vi "LinearQuadraticRegulator_LatencyCompensate.vi"(8 "InputDelay_Seconds":dbl, 9 "dT_Seconds":dbl, 10 "Plant":T1, 11 "in LinearQuadraticRegulator":T3) -> (0 "Error":bool, 3 "out LinearQuadraticRegulator":T3, 4 "ExponentNotRational":bool)   [LabVIEW 2019, in "Trajectory_Library.lvlib"]
doc: "Adjusts LQR controller gain to compensate for a pure time delay in the input.\n \nLinear-Quadratic regulator controller gains tend to be aggressive. If sensor measurements are time-delayed too long, the LQR may be unstable. However, if we know the amount of delay, we can compute the control based on where the system will be after the time delay.\n \nSee https://file.tavsys.net/control/controls-engineering-in-frc.pdf appendix C.4 for a derivation.\n \nInputs:\n - inLinearQuadraticRegulator -- controller data cluster\n - plant -- The plant being controlled.\n - dtSeconds -- Discretization timestep in seconds.\n - inputDelaySeconds -- Input time delay in seconds.\n\nOutput:\n - outLinearQuadraticRegulator -- updated data cluster\n - error -- If TRUE, an error occured.\n - exponentNotRational -- if TRUE, an error occured."
uses:
  Trajectory_Library.lvlib
  TypeDef/LINEAR_QUADRATIC_REGULATOR.ctl
  <vilib>/Analysis/Matrix/Datatypes/RealMatrix.ctl
  TypeDef/LINEAR_SYSTEM.ctl
  <vilib>/Analysis/baseanly.llb/Real A x B.vi
  MatrixHelper_CoerceSize.vi
  MatBuilder_Create.vi
  Matrix_Exp.vi
  Matrix_AssignBlock.vi
  Matrix_ExtractFrom.vi
  <vilib>/Analysis/7linalg.llb/Matrix Power.vi
  <vilib>/Analysis/7linalg.llb/Real Matrix Power.vi
  <vilib>/Analysis/7linalg.llb/Matrix Exp.vi
  <vilib>/Analysis/7linalg.llb/Real Matrix Exp.vi
  <vilib>/Analysis/Matrix/Numeric/Multiply/Multiply.vi
  <vilib>/Analysis/Matrix/Numeric/Multiply/Multiply - RM,R.vi
  <vilib>/Analysis/Matrix/Numeric/Subtract/Subtract - RM,RM.vi
  <vilib>/Analysis/7linalg.llb/Matrix Logarithm.vi
  <vilib>/Analysis/7linalg.llb/Real Matrix Logarithm.vi
  <vilib>/Analysis/Matrix/Numeric/Complex/Complex To Cartesian.vi
  <vilib>/Analysis/Matrix/Numeric/Complex/Complex To Cartesian - CM.vi
  <vilib>/Analysis/NI_AALBase.lvlib
  <vilib>/Analysis/Matrix/NI_Matrix.lvlib
panel:
  # "<States,States>"
  # "<States,Inputs>"
  # "<Outputs,States>"
  # "<Outputs,Inputs>"
  # "Ref State <States,1>"
  # "Comp and capped \noutput <Inputs,1>"
  # "Controller gain\n<Inputs,States>"
  # "Ref State <States,1>"
  # "Comp and capped \noutput <Inputs,1>"
  # "Controller gain\n<Inputs,States>"
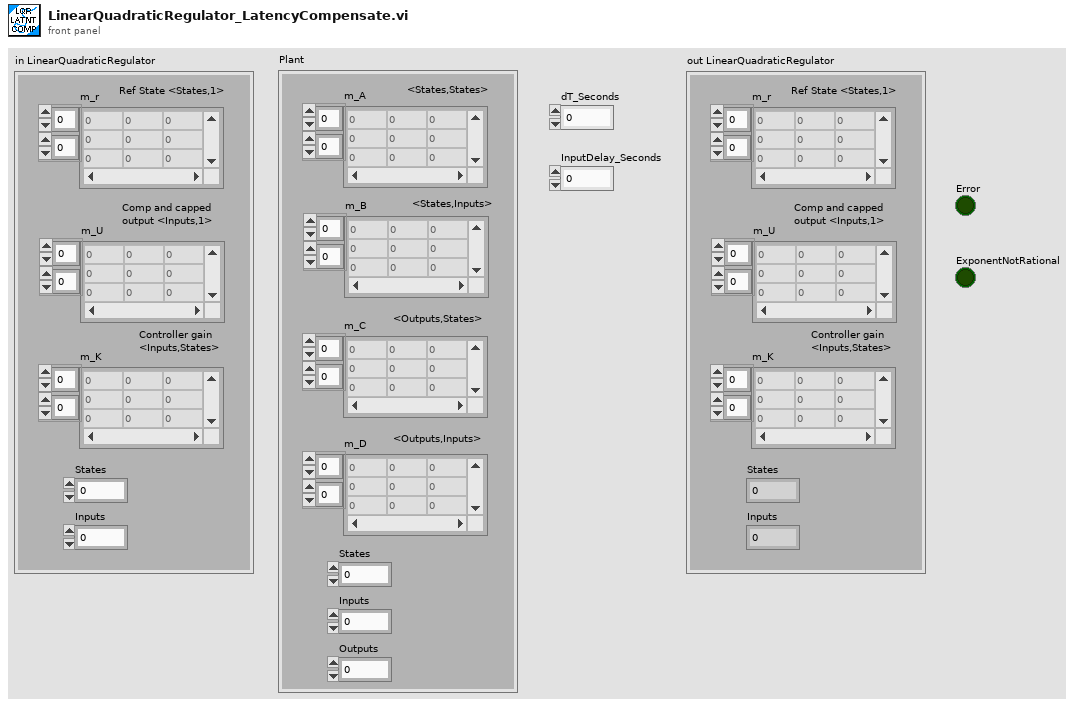
[diagram p1: front panel]
types:
  T1 = typedef "Trajectory_Library.lvlib/LINEAR_SYSTEM.ctl" = cluster{"m_A":T2, "m_B":T2, "m_C":T2, "m_D":T2, "States":i32, "Inputs":i32, "Outputs":i32}
  T2 = typedef "NI_Matrix.lvlib/RealMatrix.ctl" = dbl[][]
  T3 = typedef "Trajectory_Library.lvlib/LINEAR_QUADRATIC_REGULATOR.ctl" = cluster{"m_r":T2, "m_U":T2, "m_K":T2, "States":i32, "Inputs":i32}
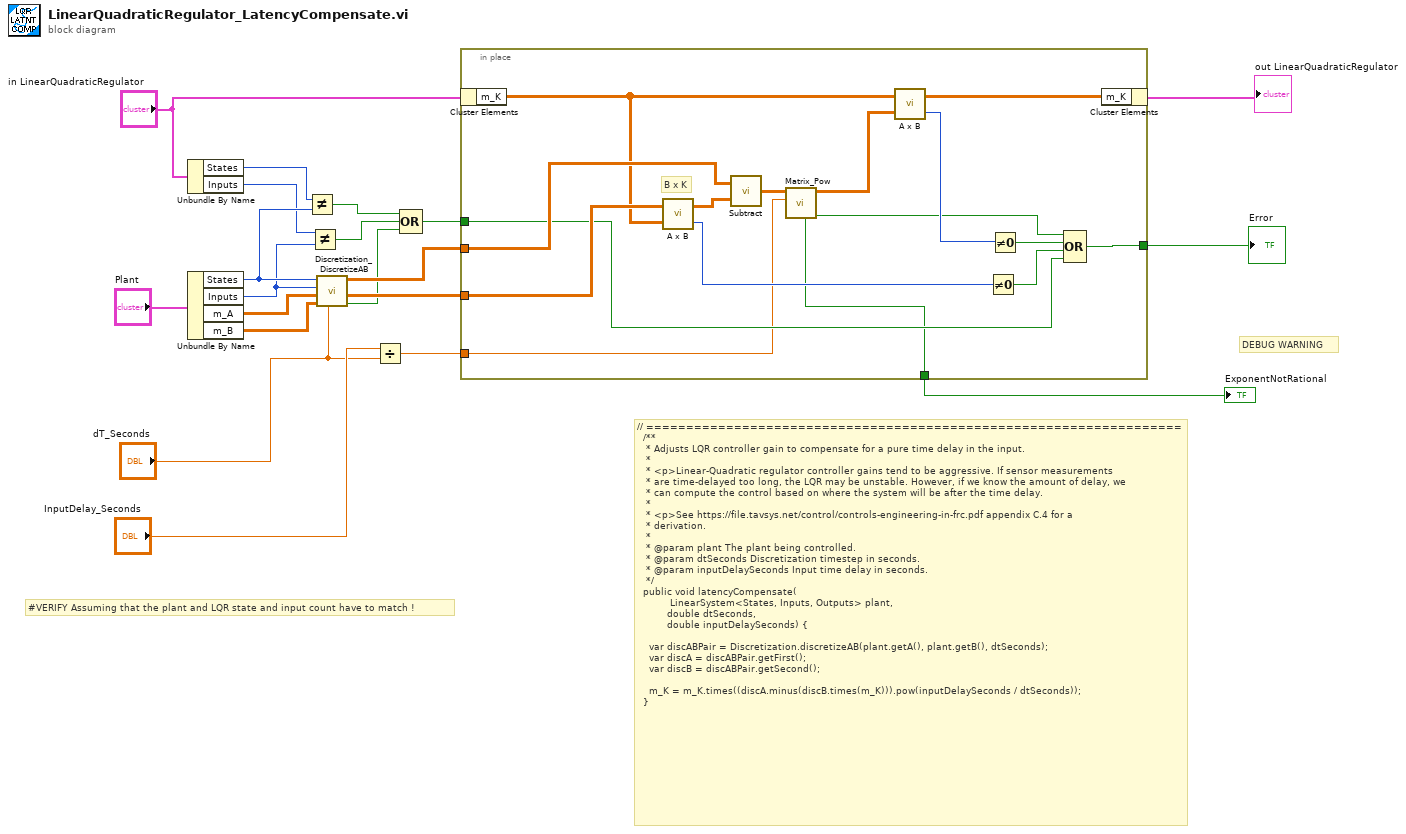
[diagram p0: block diagram]
diagram:
  # "DEBUG WARNING"
  # "#VERIFY Assuming that the plant and LQR state and input count have to match !"
  # "// ===================================================================\n  /**\n   * Adjusts LQR controller gain to compensate for a pure time delay in the input.\n   *\n   * <p>Linear-Quadratic regulator controller gains tend to be aggressive. If sensor measurements\n   * are time-delayed too long, the LQR may be unstable. However, if we know the amount of delay, we\n   * can compute the control based on where the system will be after the time delay.\n   *\n   * <p>See https://file.tavsys.net/control/controls-engineering-in-frc.pdf appendix C.4 for a\n   * derivation.\n   *\n   * @param plant The plant being controlled.\n   * @param dtSeconds Discretization timestep in seconds.\n   * @param inputDelaySeconds Input time delay in seconds.\n   */\n  public void latencyCompensate(\n          \tLinearSystem<States, Inputs, Outputs> plant, \n\t         double dtSeconds, \n\t         double inputDelaySeconds) {\n\n    var discABPair = Discretization.discretizeAB(plant.getA(), plant.getB(), dtSeconds);\n    var discA = discABPair.getFirst();\n    var discB = discABPair.getSecond();\n\n    m_K = m_K.times((discA.minus(discB.times(m_K))).pow(inputDelaySeconds / dtSeconds));\n  }"
  n1 = Unbundle By Name("in LinearQuadraticRegulator") -> ("States"=w11:i32, "Inputs"=w9:i32)
  n2 = Unbundle By Name("Plant") -> ("States"=w10:i32, "Inputs"=w8:i32, "m_A"=w17:T2, "m_B"=w16:T2)
  n3 = Not Equal?(x=w11, y=w10) -> (x != y?=w6:bool)
  n4 = Not Equal?(x=w9, y=w8) -> (x != y?=w5:bool)
  n5 = call "Discretization_DiscretizeAB.vi"("dT_Seconds"="dT_Seconds", "ContB"=w16, "ContA"=w17, "Inputs"=w8, "States"=w10) -> ("Error"=w1:bool, "DiscB"=w14:T2, "DiscA"=w15:T2)  [unwired: 4 in]
  n6 = Divide(x="InputDelay_Seconds", y="dT_Seconds") -> (x/y=w7:dbl)
  n7 = Compound Arithmetic op=OR(w6, w5, w1) -> (w4:bool)
  n8 = in-place {
    in-place-border: w15 -> [w34]
    in-place-border: w14 -> [w36]
    in-place-border: w7 -> [w25]
    in-place-border: w4 -> [w29]
    in-place-border: [w28] -> w3
    in-place-border: [w26] -> w2
    # "B x K"
    n9 = in-place-cluster #1("in LinearQuadraticRegulator") -> ("m_K"=w23:T2)
    n10 = call-poly <vilib>:"A x B.vi"("B"=w23, "A"=w36) -> ("error"=w32:i32, "A x B"=w35:T2)
    n11 = call-poly <vilib>:"Subtract.vi"("Real Matrix B"=w35, "Real Matrix A"=w34) -> ("A - B"=w24:T2)
    n12 = call "Matrix_Pow.vi"("Exponent"=w25, "input matrix"=w24) -> ("Error"=w27:bool, "output matrix"=w22:T2, "ExponentNotRational"=w26:bool)  [unwired: 7 in]
    n13 = call-poly <vilib>:"A x B.vi"("B"=w22, "A"=w23) -> ("error"=w33:i32, "A x B"=w21:T2)
    n14 = Not Equal To 0?(x=w32) -> (x != 0?=w30:bool)
    n15 = Not Equal To 0?(x=w33) -> (x != 0?=w31:bool)
    n16 = Compound Arithmetic op=OR(w27, w31, w30, w29) -> (w28:bool)
    n17 = in-place-cluster #1("m_K"=w21) -> (→"out LinearQuadraticRegulator":T3)
  }
  "Error" <- w3
  "ExponentNotRational" <- w2
